vi "Decide next action Rate base.vi"(8 "error in (no error)":errorcluster, 9 "Seek?":bool, 10 "Seek positive polarization?":bool, 11 "Automation in":refnum<class "Automation.lvclass">) -> (0 "error out":errorcluster, 1 "Should reseek?":bool, 2 "Decision":T1, 3 "Automation out":refnum<class "Automation.lvclass">)   [LabVIEW 2019, in "Automation.lvclass"]
uses:
  Automation.lvclass
  Automatic mode/Controller decision.ctl
  Automation.lvclass/Automation.ctl
  <vilib>/gmath/NI_Gmath.lvlib
panel:
  out "T2":dbl
  out "T1":dbl
  out "Polarizations":dbl[](array[numeric])
  out "x-y":dbl
  out "Slope 2":dbl
  out "Slope 1":dbl
  out "spread value":dbl
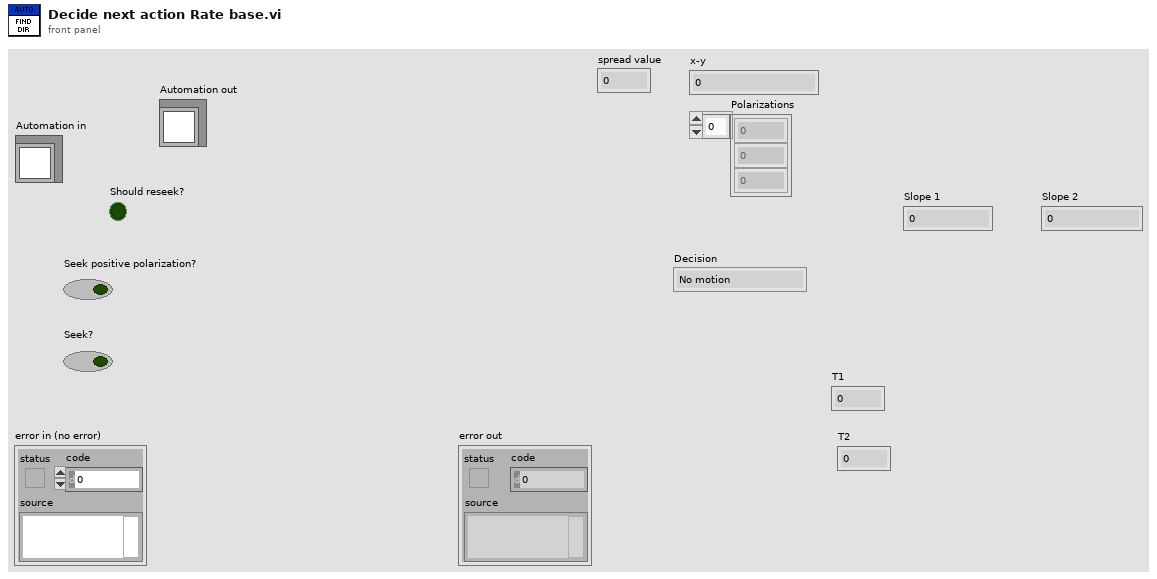
[diagram p1: front panel]
types:
  T1 = typedef "Controller decision.ctl" = enum16{"No motion", "Switch direction", "Keep current direction"}
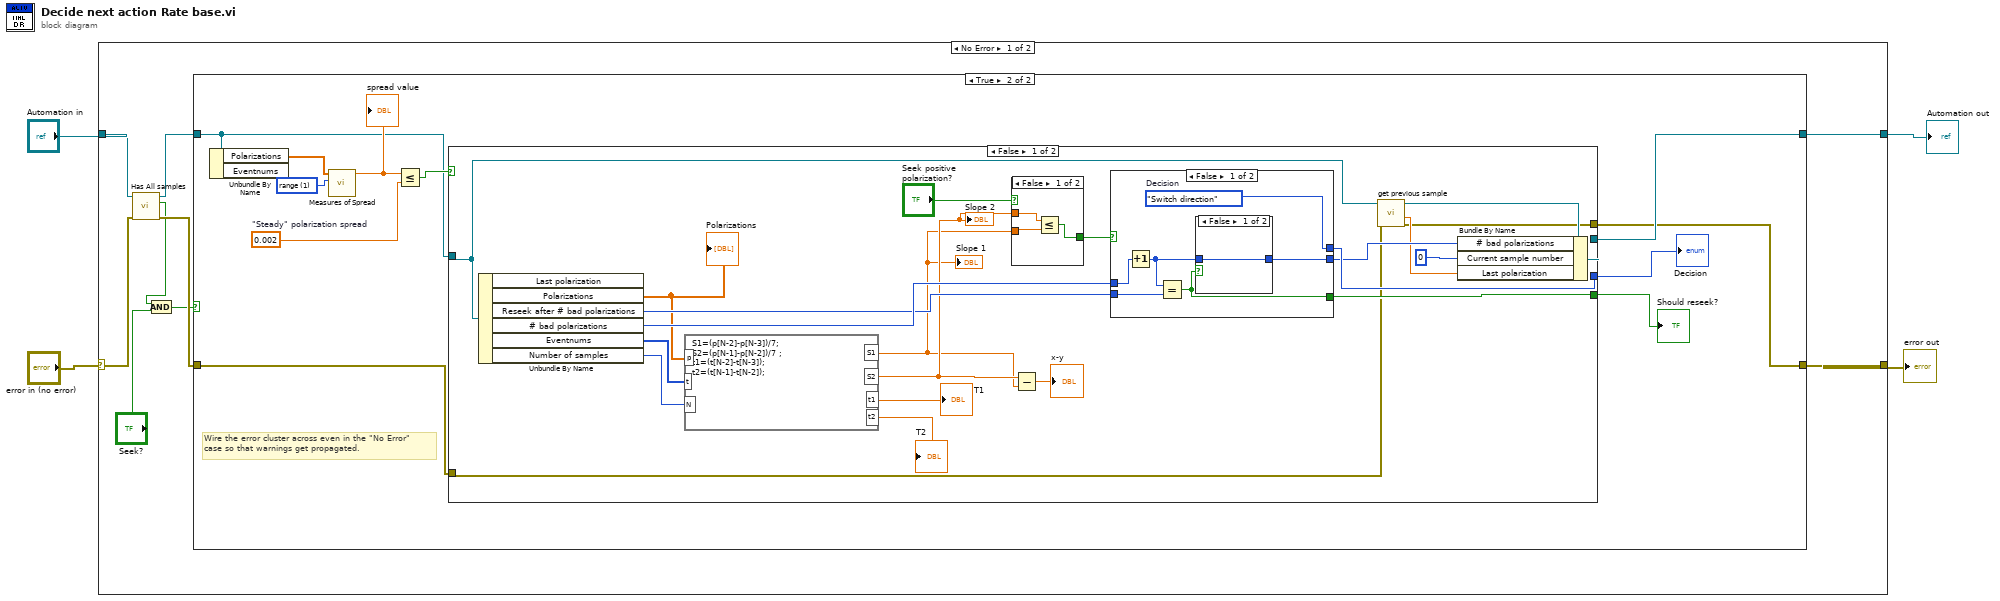
[diagram p0: block diagram]
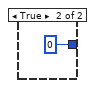
[diagram p3: hidden frame]
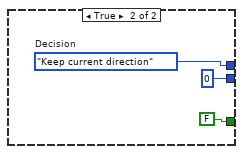
[diagram p4: hidden frame]
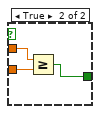
[diagram p5: hidden frame]
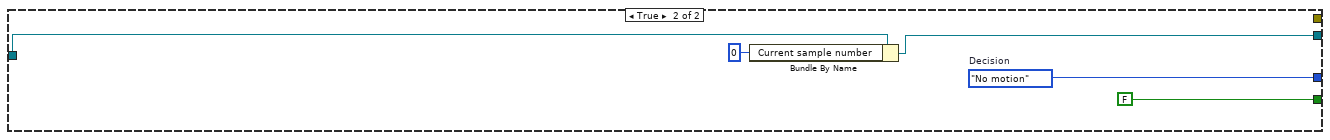
[diagram p6: hidden frame]
diagram:
  n1 = case shown="No Error" "error in (no error)" {
    selector: "error in (no error)" -> [w10 w72]
    tunnel: [w12 w72] -> w3
    tunnel: [w13 w71] -> w1
    tunnel: "Automation in" -> [w11 w71]
    frame No Error {
      n2 = call "Has All samples.vi"("error in (no error)"=w10, "Automation in"=w11) -> ("error out"=w9:errorcluster, "Has all samples?"=w6:bool, "Automation out"=w8:refnum<class "Automation.lvclass">)  [unwired: 7 in]
      n3 = And(x=w6, y="Seek?") -> (x .and. y?=w7:bool)
      n4 = case shown="True" w7 {
        tunnel: w8 -> [w14 w22]
        tunnel: [w14 w20] -> w13
        tunnel: [w15 w17] -> w12
        tunnel: w9 -> [w15 w16]
        frame False {
        }
        frame True {
          w24 = 0.002  # "Steady" polarization spread
          w26 = 1 items=["standard deviation", "range", "mean absolute deviation", "interquartile range"] ("type")
          # "Wire the error cluster across even in the \"No Error\"\ncase so that warnings get propagated."
          n5 = Unbundle By Name(w22) -> ("Polarizations"=w21:dbl[])  [unwired: 1 out]
          n6 = call <vilib>:"Measures of Spread.vi"("type"=w26, "x array"=w21) -> ("spread value"=w25:dbl)  [unwired: 8 in, 1 out]
          "spread value" <- w25
          n7 = Less Or Equal?(x=w25, y=w24) -> (x <= y?=w23:bool)
          n8 = case shown="False" w23 {
            tunnel: [w44 w67] -> w20
            tunnel: [w48 w69] -> w19
            tunnel: [w45 FALSE] -> w18
            tunnel: w22 -> [w41 w68]
            tunnel: [w38 _] -> w17
            tunnel: w16 -> [w37 _]
            frame False {
              n9 = Unbundle By Name(w41) -> ("Polarizations"=w36:dbl[], "Reseek after # bad polarizations"=w43:u32, "# bad polarizations"=w46:u32, "Eventnums"=w35:i64[], "Number of samples"=w34:i32)  [unwired: 1 out]
              "Polarizations" <- w36
              n10 = formula code="S1=(p[N-2]-p[N-3])/7;\nS2=(p[N-1]-p[N-2])/7 ;\nt1=(t[N-2]-t[N-3]);\nt2=(t[N-1]-t[N-2]);"("p"=w36, "t"=w35, "N"=w34) -> ("S1"=w29:dbl, "S2"=w30:dbl, "t1"=→"T1":dbl, "t2"=→"T2":dbl)
              "Slope 1" <- w29
              "Slope 2" <- w30
              n11 = case shown="False" "Seek positive polarization?" {
                tunnel: [w62 w65] -> w32
                tunnel: w30 -> [w61 w64]
                tunnel: w29 -> [w60 w63]
                frame False {
                  n12 = Less Or Equal?(x=w61, y=w60) -> (x <= y?=w62:bool)
                }
                frame True {
                  n13 = Greater Or Equal?(x=w64, y=w63) -> (x >= y?=w65:bool)
                }
              }
              n14 = Subtract(x=w30, y=w29) -> (x-y=→"x-y":dbl)
              n15 = case shown="False" w32 {
                tunnel: [w49 w57] -> w48
                tunnel: [w51 u32 0] -> w47
                tunnel: w46 -> [w54 _]
                tunnel: [w52 FALSE] -> w45
                tunnel: w43 -> [w53 _]
                frame False {
                  w49 = Controller_decision."Switch direction"  # Decision
                  n16 = Increment(x=w54) -> (x+1=w50:u32)
                  n17 = Equal?(x=w50, y=w53) -> (x = y?=w52:bool)
                  n18 = case shown="False" w52 {
                    tunnel: [w55 0] -> w51
                    tunnel: w50 -> [w55 _]
                    frame False {
                    }
                    frame True {
                    }
                  }
                }
                frame True {
                  w57 = Controller_decision."Keep current direction"  # Decision
                }
              }
              n19 = call "get previous sample.vi"("error in (no error)"=w37, "Automation in"=w41) -> ("error out"=w38:errorcluster, "Polarization"=w39:dbl, "Automation out"=w40:refnum<class "Automation.lvclass">)  [unwired: 6 in, 1 out]
              n20 = Bundle By Name(cluster=w40, "# bad polarizations"=w47, "Current sample number"=0, "Last polarization"=w39) -> (w44:refnum<class "Automation.lvclass">)
            }
            frame True {
              w69 = Controller_decision."No motion"  # Decision
              n21 = Bundle By Name(cluster=w68, "Current sample number"=0) -> (w67:refnum<class "Automation.lvclass">)
            }
          }
          "Decision" <- w19
          "Should reseek?" <- w18
        }
      }
    }
    frame Error {
    }
  }
  "error out" <- w3
  "Automation out" <- w1
